vi "Init.vi"(8 "error in (no error)":errorcluster) -> (0 "error out":errorcluster, 2 "Propeller":refnum<vi>, 3 "Scene Object Out":refnum<vi>)   [LabVIEW 2013]
uses:
  <vilib>/picture/3D Picture Control/Object/Create Object (drawable).vi
  <vilib>/picture/3D Picture Control/Object/Create Object (name).vi
  <vilib>/picture/3D Picture Control/Helpers/Apply Texture (no reference).vi
  <vilib>/picture/3D Picture Control/Object/Add Object (no reference).vi
  <vilib>/picture/3D Picture Control/Object/Add Object (reference).vi
  <vilib>/picture/3D Picture Control/NI_3D Picture Control.lvlib
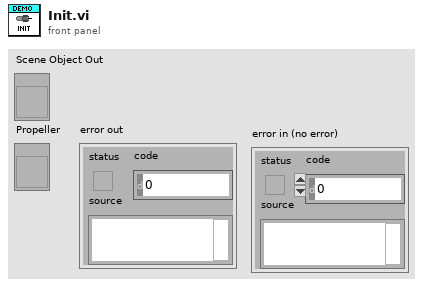
[diagram p1: front panel]
types:
  T1 = enum16{"As a Decal", "With Modulation", "With Blending", "As a replacement"}
  T2 = typedef "imagedata.ctl" = cluster{"image type":i32, "image depth":i32, "image":u8[], "mask":u8[], "colors":u32[], "Rectangle":cluster{"left":i16, "top":i16, "right":i16, "bottom":i16}}
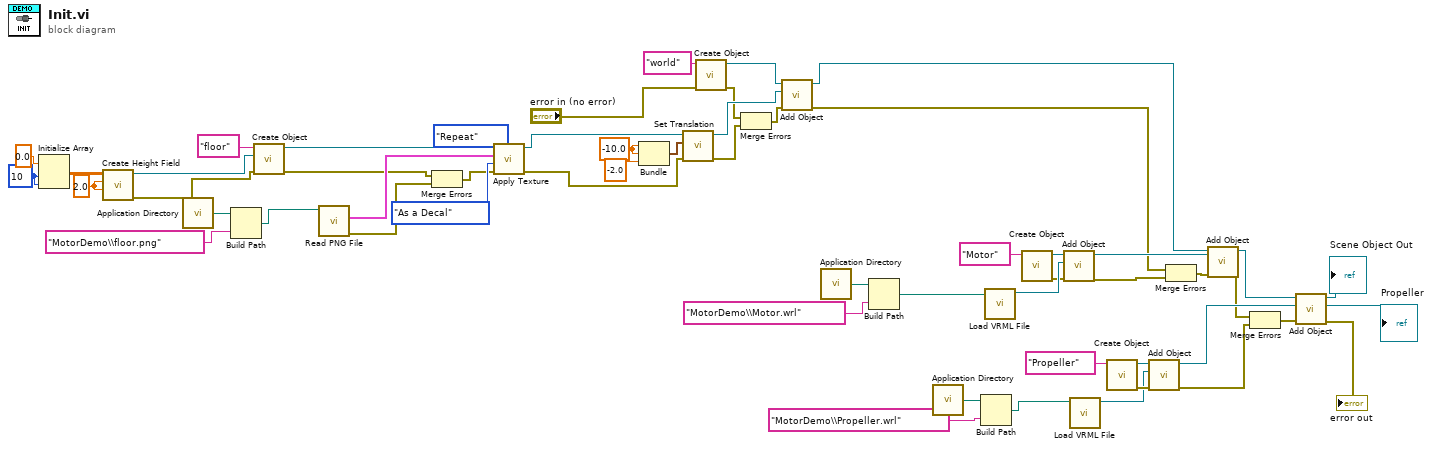
[diagram p0: block diagram]
diagram:
  w52 = 10 ("dimension size")
  w53 = sgl -10.0 ("y")
  w55 = sgl 2.0 ("Row Interval")
  n1 = Initialize Array(0.0 ("element"), w52, w52) -> (w50:dbl[][])
  n2 = call <vilib>:"Create Height Field.vi"("Column Interval"=w55, "Row Interval"=w55, "Data"=w50) -> ("error out"=w32:errorcluster, "New Height Field Refnum"=w43:refnum<vi>)  [unwired: 1 in, 6 out]
  n3 = call <vilib>:"Application Directory.vi"() -> ("Application Directory"=w8:path)
  n4 = Build Path(base path=w8, name or relative path="MotorDemo\\floor.png") -> (appended path=w9:path)
  n5 = call-poly <vilib>:"Create Object.vi"("error in (no error)"=w32, "Geometry"=w43, "Name"="floor") -> ("error out"=w33:errorcluster, "Scene:New Object"=w46:refnum<vi>)  [unwired: 7 in]
  n6 = call <vilib>:"Read PNG File.vi"("path to PNG file"=w9) -> ("error out"=w35:errorcluster, "image data"=w44:T2)  [unwired: 1 in, 8 out]
  n7 = Merge Errors(w33, w35) -> (w34:errorcluster)
  n8 = call-poly <vilib>:"Apply Texture.vi"("Horizontal Wrap Mode"=enum16{"Clamp", "Repeat"}."Repeat", "error in (no error)"=w34, "Apply Mode"=T1."As a Decal", "Image Data"=w44, "Scene Object In"=w46) -> ("error out"=w36:errorcluster, "Scene Object Out"=w48:refnum<vi>)  [unwired: 5 in]
  n9 = Bundle("y"=w53, "y"=w53, "-x"=-2.0) -> (w54:cluster{"y":sgl, "y":sgl, "-x":dbl})  [unwired: 1 out]
  n10 = call <vilib>:"Set Translation.vi"("error in (no error)"=w36, "Translation"=w54, "Scene Object"=w48) -> ("error out"=w37:errorcluster, "Translated Object"=w41:refnum<vi>)  [unwired: 7 out]
  n11 = call-poly <vilib>:"Create Object.vi"("error in (no error)"="error in (no error)", "Name"="world") -> ("error out"=w39:errorcluster, "Scene:New Object"=w40:refnum<vi>)  [unwired: 8 in]
  n12 = Merge Errors(w39, w37) -> (w38:errorcluster)
  n13 = call-poly <vilib>:"Add Object.vi"("error in (no error)"=w38, "New Object In"=w41, "Scene Object In"=w40) -> ("error out"=w10:errorcluster, "Scene Object Out"=w11:refnum<vi>)  [unwired: 7 in]
  n14 = call <vilib>:"Application Directory.vi"() -> ("Application Directory"=w6:path)
  n15 = Build Path(base path=w6, name or relative path="MotorDemo\\Motor.wrl") -> (appended path=w4:path)
  n16 = call <vilib>:"Application Directory.vi"() -> ("Application Directory"=w2:path)
  n17 = Build Path(base path=w2, name or relative path="MotorDemo\\Propeller.wrl") -> (appended path=w1:path)
  n18 = call <vilib>:"Load VRML File.vi"("Path"=w4) -> ("Scene:Read Scene File"=w29:refnum<vi>)  [unwired: 9 in, 1 out]
  n19 = call-poly <vilib>:"Create Object.vi"("Name"="Motor") -> ("error out"=w27:errorcluster, "Scene:New Object"=w30:refnum<vi>)  [unwired: 9 in]
  n20 = call-poly <vilib>:"Add Object.vi"("error in (no error)"=w27, "New Object In"=w29, "Scene Object In"=w30) -> ("error out"=w20:errorcluster, "Scene Object Out"=w19:refnum<vi>)  [unwired: 7 in]
  n21 = call <vilib>:"Load VRML File.vi"("Path"=w1) -> ("Scene:Read Scene File"=w23:refnum<vi>)  [unwired: 9 in, 1 out]
  n22 = call-poly <vilib>:"Create Object.vi"("Name"="Propeller") -> ("error out"=w25:errorcluster, "Scene:New Object"=w22:refnum<vi>)  [unwired: 9 in]
  n23 = call-poly <vilib>:"Add Object.vi"("error in (no error)"=w25, "New Object In"=w23, "Scene Object In"=w22) -> ("error out"=w15:errorcluster, "Scene Object Out"=w18:refnum<vi>)  [unwired: 7 in]
  n24 = Merge Errors(w10, w20) -> (w26:errorcluster)
  n25 = call-poly <vilib>:"Add Object.vi"("error in (no error)"=w26, "New Object In"=w19, "Scene Object In"=w11) -> ("error out"=w16:errorcluster, "Scene Object Out"=w21:refnum<vi>)  [unwired: 7 in]
  n26 = Merge Errors(w16, w15) -> (w17:errorcluster)
  n27 = call-poly <vilib>:"Add Object.vi"("error in (no error)"=w17, "New Object In"=w18, "Scene Object In"=w21) -> ("error out"=→"error out":errorcluster, "New Object Out"=→"Propeller":refnum<vi>, "Scene Object Out"=→"Scene Object Out":refnum<vi>)  [unwired: 6 in]
